vi "Clear References.vi"(8 "error in (no error)":errorcluster, 11 "References":T1) -> (0 "error out":errorcluster)   [LabVIEW 2019, in "Lock Library.lvlib"]
uses:
  Lock Library.lvlib
  References.ctl
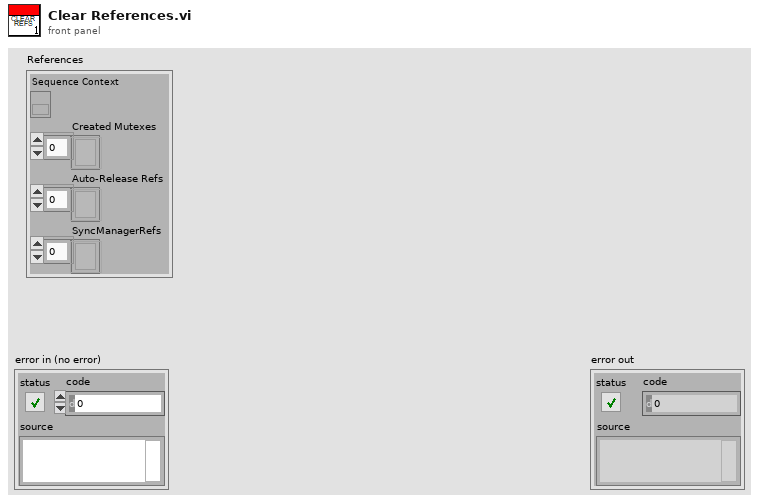
[diagram p1: front panel]
types:
  T1 = typedef "Lock Library.lvlib/References.ctl" = cluster{"Sequence Context":refnum<k7>, "Created Mutexes":refnum<k7>[], "Auto-Release Refs":refnum<k7>[], "SyncManagerRefs":refnum<k7>[]}
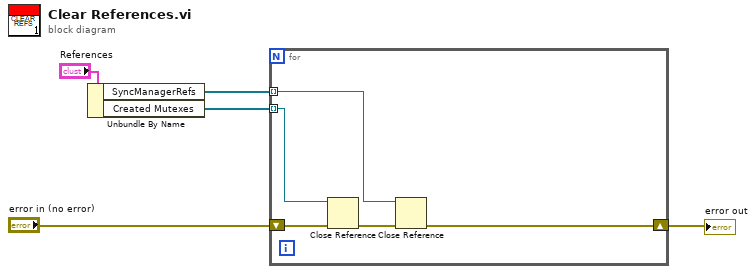
[diagram p0: block diagram]
diagram:
  n1 = Unbundle By Name("References") -> ("SyncManagerRefs"=w3:refnum<k7>[], "Created Mutexes"=w2:refnum<k7>[])
  n2 = for {
    shift-right: [w6] -> w1
    shift-left: "error in (no error)" -> [w10]
    tunnel: w3 -> [w8] mode=indexing
    tunnel: w2 -> [w9] mode=indexing
    n3 = Close Reference(reference=w9, error in (no error)=w10) -> (error out=w7:errorcluster)
    n4 = Close Reference(reference=w8, error in (no error)=w7) -> (error out=w6:errorcluster)
  }
  "error out" <- w1
